vi "Update Wfm Grp Ctrls.vi"(8 "error in (no error)":errorcluster, 10 "Wfm Grp Data":T2, 11 "Ctrl Refs":T1) -> (0 "error out":errorcluster)   [LabVIEW 2025, in "TDMS Waveform Creator UI.lvlib"]
uses:
  TDMS Waveform Creator UI.lvlib
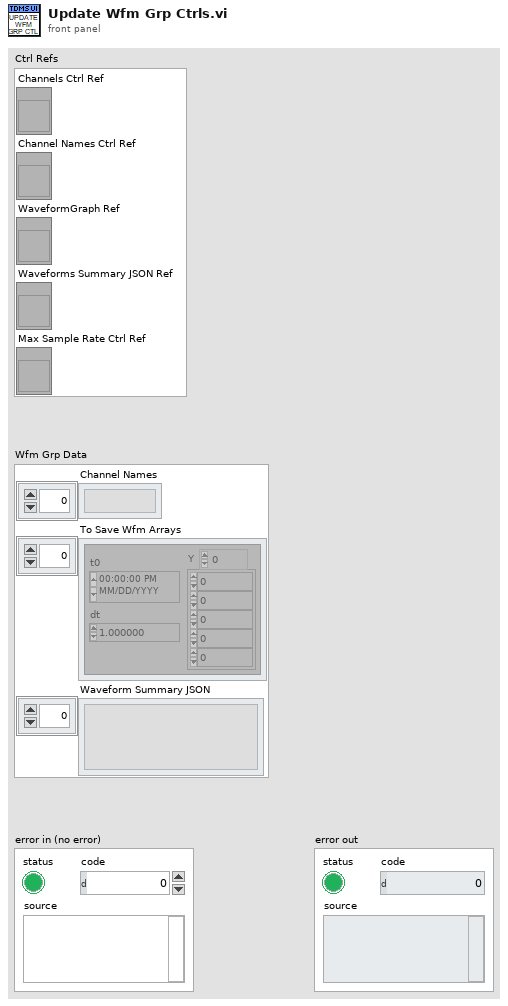
[diagram p1: front panel]
types:
  T1 = cluster{"Channels Ctrl Ref":refnum<vi>, "Channel Names Ctrl Ref":refnum<vi>, "WaveformGraph Ref":refnum<vi>, "Waveforms Summary JSON Ref":refnum<vi>, "Max Sample Rate Ctrl Ref":refnum<vi>}
  T2 = cluster{"Channel Names":string[], "To Save Wfm Arrays":waveform(dbl)[], "Waveform Summary JSON":string[]}
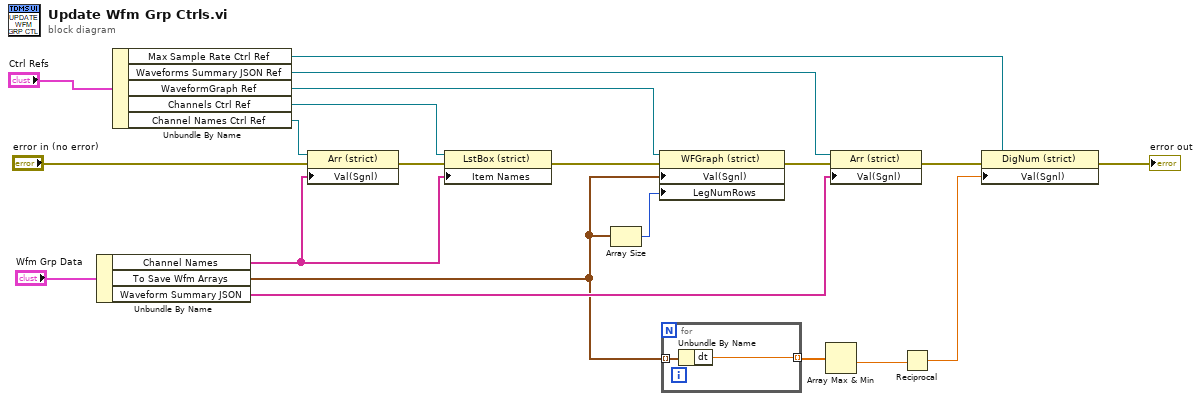
[diagram p0: block diagram]
diagram:
  n1 = Unbundle By Name("Wfm Grp Data") -> ("Channel Names"=w1:string[], "To Save Wfm Arrays"=w7:waveform(dbl)[], "Waveform Summary JSON"=w11:string[])
  n2 = Unbundle By Name("Ctrl Refs") -> ("Max Sample Rate Ctrl Ref"=w8:refnum<vi>, "Waveforms Summary JSON Ref"=w13:refnum<vi>, "WaveformGraph Ref"=w14:refnum<vi>, "Channels Ctrl Ref"=w2:refnum<vi>, "Channel Names Ctrl Ref"=w15:refnum<vi>)
  n3 = property on="Property Node" class="Arr (strict)"(reference=w15, error in="error in (no error)", "Val(Sgnl)"=w1) -> (error out=w20:errorcluster)  [unwired: 1 out]
  n4 = property class="LstBox (strict)"(reference=w2, error in=w20, "Item Names"=w1) -> (error out=w3:errorcluster)  [unwired: 1 out]
  n5 = Array Size(array=w7) -> (size(s)=w18:i32)
  n6 = property on="Property Node" class="WFGraph (strict)"(reference=w14, error in=w3, "Val(Sgnl)"=w7, "LegNumRows"=w18) -> (error out=w12:errorcluster)  [unwired: 1 out]
  n7 = for {
    tunnel: w7 -> [w22] mode=indexing
    tunnel: [w21] -> w6 mode=indexing
    n8 = Unbundle By Name(w22) -> ("dt"=w21:dbl)
  }
  n9 = Array Max & Min(array=w6) -> (min value=w5:dbl)  [unwired: 3 out]
  n10 = property on="Property Node" class="Arr (strict)"(reference=w13, error in=w12, "Val(Sgnl)"=w11) -> (error out=w10:errorcluster)  [unwired: 1 out]
  n11 = Reciprocal(x=w5) -> (1/x=w4:dbl)
  n12 = property class="DigNum (strict)"(reference=w8, error in=w10, "Val(Sgnl)"=w4) -> (error out=→"error out":errorcluster)  [unwired: 1 out]
